vi "Close.vi"(8 "error in":errorcluster, 11 "PCAN Basic in":refnum<class "PCAN Basic Base Configure Strategy.lvclass">) -> (0 "error out":errorcluster, 3 "PCAN Basic out":refnum<class "PCAN Basic Base Configure Strategy.lvclass">)   [LabVIEW 2025, in "PCAN Basic Base Configure Strategy.lvclass"]
uses:
  PCAN Basic Base Configure Strategy.lvclass
  PCAN Basic Base Configure Strategy.lvclass/PCAN Basic Base Configure Strategy.ctl
  <instrlib>/Peter/PCAN Basic/PCANBasic.lvlib
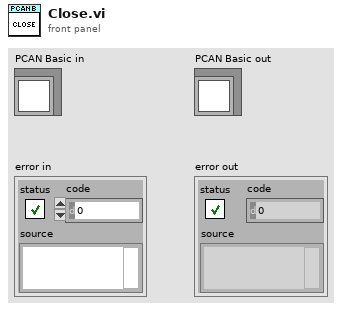
[diagram p1: front panel]
types:
  T1 = typedef "PCANBasic.lvlib/TPCANHandle.ctl" = u16
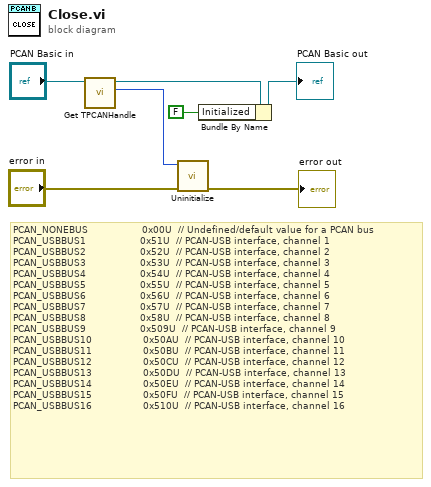
[diagram p0: block diagram]
diagram:
  # "PCAN_NONEBUS                  0x00U  // Undefined/default value for a PCAN bus\nPCAN_USBBUS1                  0x51U  // PCAN-USB interface, channel 1\nPCAN_USBBUS2                  0x52U  // PCAN-USB interface, channel 2\nPCAN_USBBUS3                  0x53U  // PCAN-USB interface, channel 3\nPCAN_USBBUS4                  0x54U  // PCAN-USB interface, channel 4\nPCAN_USBBUS5                  0x55U  // PCAN-USB interface, channel 5\nPCAN_USBBUS6                  0x56U  // PCAN-USB interface, channel 6\nPCAN_USBBUS7                  0x57U  // PCAN-USB interface, channel 7\nPCAN_USBBUS8                  0x58U  // PCAN-USB interface, channel 8\nPCAN_USBBUS9                  0x509U  // PCAN-USB interface, channel 9\nPCAN_USBBUS10                 0x50AU  // PCAN-USB interface, channel 10\nPCAN_USBBUS11                 0x50BU  // PCAN-USB interface, channel 11\nPCAN_USBBUS12                 0x50CU  // PCAN-USB interface, channel 12\nPCAN_USBBUS13                 0x50DU  // PCAN-USB interface, channel 13\nPCAN_USBBUS14                 0x50EU  // PCAN-USB interface, channel 14\nPCAN_USBBUS15                 0x50FU  // PCAN-USB interface, channel 15\nPCAN_USBBUS16                 0x510U  // PCAN-USB interface, channel 16"
  n1 = call "Get TPCANHandle.vi"("PCAN Basic Base Configure Strategy in"="PCAN Basic in") -> ("TPCANHandle"=w1:T1, "PCAN Basic Base Configure Strategy out"=w3:refnum<class "PCAN Basic Base Configure Strategy.lvclass">)  [unwired: 9 in]
  n2 = call <instrlib>:"Uninitialize.vi"("error in"="error in", "TPCANHandle in"=w1) -> ("error out"=→"error out":errorcluster)  [unwired: 8 in, 1 out]
  n3 = Bundle By Name(cluster=w3, "Initialized"=FALSE) -> (→"PCAN Basic out":refnum<class "PCAN Basic Base Configure Strategy.lvclass">)
